vi "API GET Filter Parameters.vi"(7 "Body Parameters Names":string[](array[string])=["id"], 8 "error in (no error)":errorcluster, 9 "Filter Parameters Names":T3={"Vin"="vin-k7ad0tyd", "R"="r-k7ad0z99", "L"="l-k7ad13xp", "C"="c-k7ad19ix"}, 10 "API Token":string="apitoken 2096a662-4947-42f5-97bc-84cfdf20fe4e:bc240510-8f48-43e3-889a-471659905c2e", 11 "API Endpoint Url":string="https://api.dev.enlil.io/api/v1/document_revisions/external/ALI00017/draft") -> (0 "error out":errorcluster, 3 "Parameters Values":T2, 4 "Response body":string, 5 "Responce headers":string, 6 "Body Parameters out":T1[](array[typedef]))   [LabVIEW 2017]
uses:
  Types/Parameters Names Type.ctl
  Types/Parameters Values Type.ctl
  Types/Body Parameter Type.ctl
  <vilib>/httpClient/LabVIEWHTTPClient.lvlib
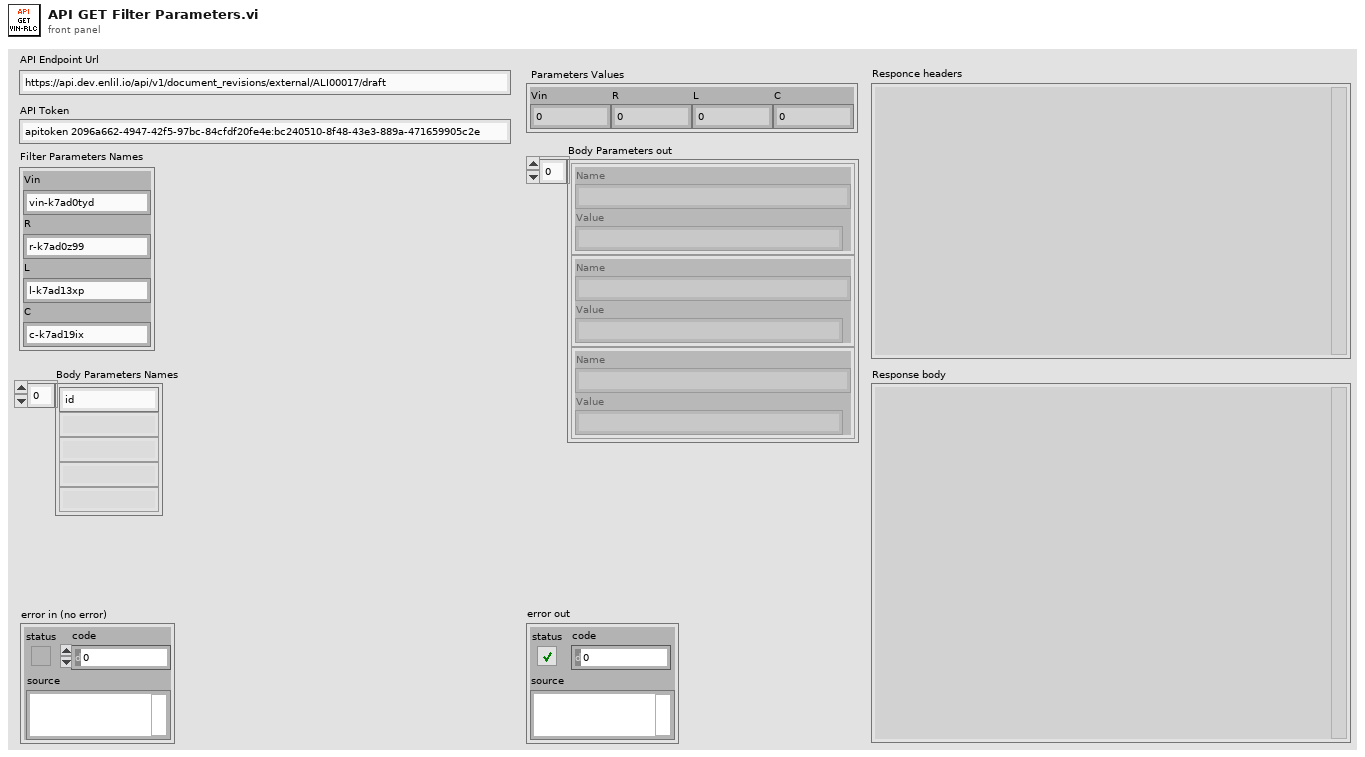
[diagram p1: front panel]
types:
  T1 = typedef "Body Parameter Type.ctl" = cluster{"Name":string, "Value":string}
  T2 = typedef "Parameters Values Type.ctl" = cluster{"Vin":dbl, "R":dbl, "L":dbl, "C":dbl}
  T3 = typedef "Parameters Names Type.ctl" = cluster{"Vin":string, "R":string, "L":string, "C":string}
  T4 = typedef "LabVIEWHTTPClient.lvlib/ClientHandle.ctl" = refnum<k1>
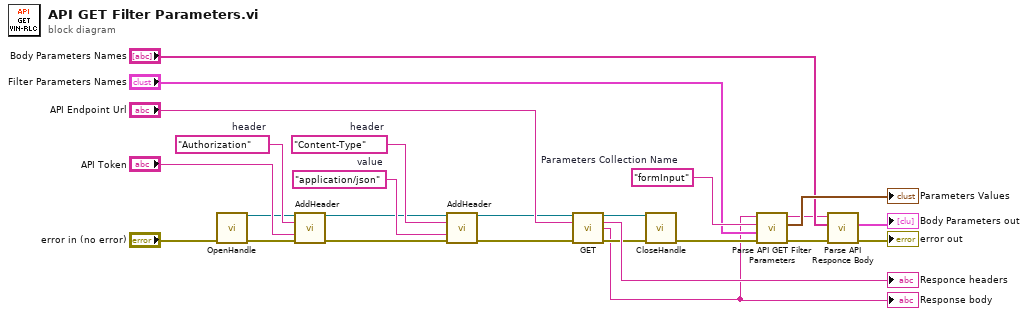
[diagram p0: block diagram]
diagram:
  w25 = "formInput"  # Parameters Collection Name
  w21 = "application/json"  # value
  w20 = "Content-Type"  # header
  w23 = "Authorization"  # header
  n1 = call <vilib>:"OpenHandle.vi"("error in (no error)"="error in (no error)") -> ("client handle out"=w7:T4, "error out"=w10:errorcluster)  [unwired: 13 in]
  n2 = call <vilib>:"AddHeader.vi"("client handle"=w7, "header"=w23, "value"="API Token", "error in (no error)"=w10) -> ("client handle out"=w8:T4, "error out"=w9:errorcluster)  [unwired: 10 in]
  n3 = call <vilib>:"AddHeader.vi"("client handle"=w8, "header"=w20, "value"=w21, "error in (no error)"=w9) -> ("client handle out"=w11:T4, "error out"=w12:errorcluster)  [unwired: 10 in]
  n4 = call <vilib>:"GET.vi"("client handle"=w11, "url"="API Endpoint Url", "error in (no error)"=w12) -> ("client handle out"=w15:T4, "headers"=→"Responce headers":string, "body"=w6:string, "error out"=w16:errorcluster)  [unwired: 9 in]
  "Response body" <- w6
  n5 = call <vilib>:"CloseHandle.vi"("client handle"=w15, "error in (no error)"=w16) -> ("error out"=w14:errorcluster)  [unwired: 13 in]
  n6 = call "Parse API GET Filter Parameters.vi"("error in (no error)"=w14, "Parameters Names"="Filter Parameters Names", "Parameters Collection Name"=w25, "Response Body in"=w6) -> ("error out"=w4:errorcluster, "Parameters Values"=→"Parameters Values":T2, "Response Body out"=w2:string)  [unwired: 5 in]
  n7 = call "Parse API Responce Body.vi"("error in (no error)"=w4, "Body Parameters Names in"="Body Parameters Names", "Response Body in"=w2) -> ("error out"=→"error out":errorcluster, "Body Parameters out"=→"Body Parameters out":T1[])  [unwired: 6 in, 1 out]
